vi "Preallocated Inverse Matrix (DBL).vi"(9 "Preallocated X":dbl[](array[numeric]), 10 "Preallocated A":dbl[](array[numeric]), 11 "Input Matrix":T1) -> (0 "error":i32, 3 "Inverse Matrix":T1)   [LabVIEW 2017, in "NI_AALPro.lvlib"]
uses:
  NI_AALPro.lvlib
  RealMatrix.ctl
  <resource>/lvanlys.dll
  NI_Matrix.lvlib
panel:
  # "Preallocated A x Vector"
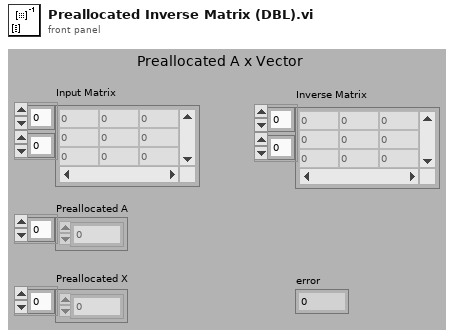
[diagram p1: front panel]
types:
  T1 = typedef "NI_Matrix.lvlib/RealMatrix.ctl" = dbl[][]
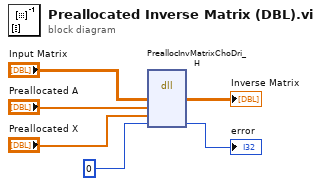
[diagram p0: block diagram]
diagram:
  n1 = dll-call lib="C:/Program Files (x86)/National Instruments/LabVIEW 2017/resource/lvanlys.*" fn="PreallocInvMatrixChoDri_H"("matrixH"="Input Matrix", "aH"="Preallocated A", "xH"="Preallocated X", "err"=0) -> ("matrixH"=→"Inverse Matrix":dbl[][], "err"=→"error":i32)  [unwired: 6 in, 2 out]
